vi "PCO_SensorInfo.vi"() -> (1 "Raw_Length":u16, 4 "Length":u16, 6 "PCO_SensorInfo_Raw_x64":T1, 7 "PCO_SensorInfo_Raw_win32":T2, 8 "PCO_SensorInfo":T3 {"iSensorInfoBits" items=["CONVERT_SENSOR_COLORIMAGE"=1, "CONVERT_SENSOR_UPPERALIGNED"=2]})   [LabVIEW 2019, in "Convert.lvlib"]
doc: "Use this template to build a VI to use as a subVI."
uses:
  Convert.lvlib
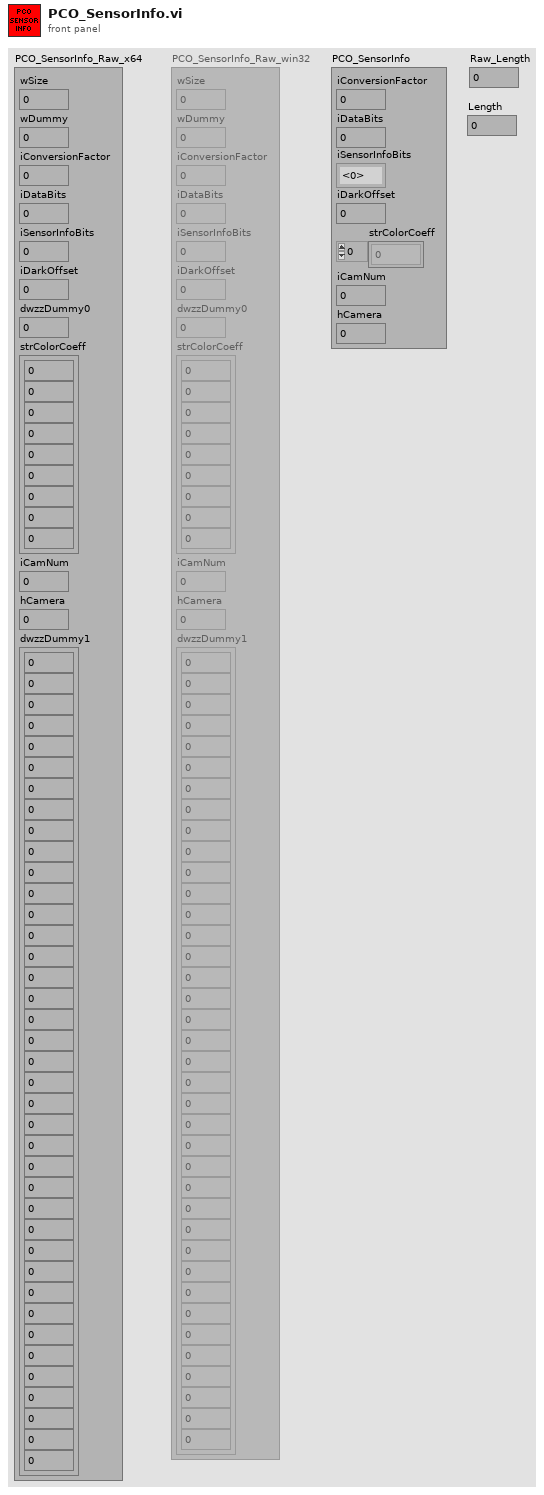
[diagram p1: front panel]
types:
  T1 = cluster{"wSize":u16, "wDummy":u16, "iConversionFactor":i32, "iDataBits":i32, "iSensorInfoBits":i32, "iDarkOffset":i32, "dwzzDummy0":u32, "strColorCoeff":cluster{dbl, dbl, dbl, dbl, dbl, dbl, dbl, dbl, dbl}, "iCamNum":i32, "hCamera":u64, "dwzzDummy1":cluster{u32, u32, u32, u32, u32, u32, u32, u32, u32, u32, u32, u32, u32, u32, u32, u32, u32, u32, u32, u32, u32, u32, u32, u32, u32, u32, u32, u32, u32, u32, u32, u32, u32, u32, u32, u32, u32, u32, u32}}
  T2 = cluster{"wSize":u16, "wDummy":u16, "iConversionFactor":i32, "iDataBits":i32, "iSensorInfoBits":i32, "iDarkOffset":i32, "dwzzDummy0":u32, "strColorCoeff":cluster{dbl, dbl, dbl, dbl, dbl, dbl, dbl, dbl, dbl}, "iCamNum":i32, "hCamera":u32, "dwzzDummy1":cluster{u32, u32, u32, u32, u32, u32, u32, u32, u32, u32, u32, u32, u32, u32, u32, u32, u32, u32, u32, u32, u32, u32, u32, u32, u32, u32, u32, u32, u32, u32, u32, u32, u32, u32, u32, u32, u32, u32}}
  T3 = cluster{"iConversionFactor":i32, "iDataBits":i32, "iSensorInfoBits":i32, "iDarkOffset":i32, "strColorCoeff":dbl[], "iCamNum":i32, "hCamera":u64}
  T4 = cluster{dbl, dbl, dbl, dbl, dbl, dbl, dbl, dbl, dbl}
  T5 = cluster{u32, u32, u32, u32, u32, u32, u32, u32, u32, u32, u32, u32, u32, u32, u32, u32, u32, u32, u32, u32, u32, u32, u32, u32, u32, u32, u32, u32, u32, u32, u32, u32, u32, u32, u32, u32, u32, u32, u32}
  T6 = cluster{u32, u32, u32, u32, u32, u32, u32, u32, u32, u32, u32, u32, u32, u32, u32, u32, u32, u32, u32, u32, u32, u32, u32, u32, u32, u32, u32, u32, u32, u32, u32, u32, u32, u32, u32, u32, u32, u32}
  T7 = enum8{"Enabled", "Disabled", "Disabled and Grayed Out"}
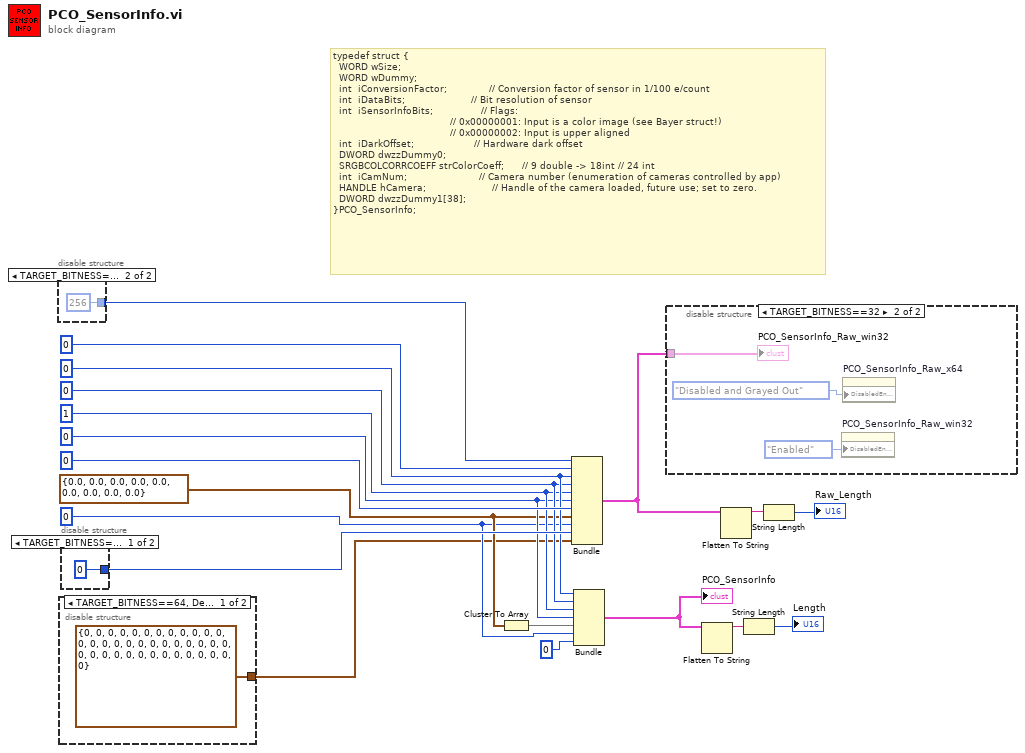
[diagram p0: block diagram]
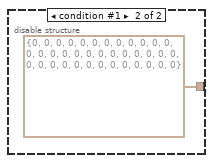
[diagram p2: hidden frame]
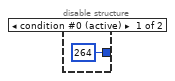
[diagram p3: hidden frame]
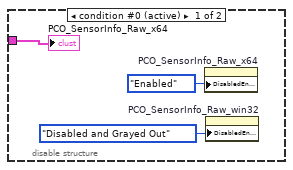
[diagram p4: hidden frame]
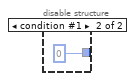
[diagram p5: hidden frame]
diagram:
  w5 = 0 ("iCamNum")
  w7 = T4 {0.0, 0.0, 0.0, 0.0, 0.0, 0.0, 0.0, 0.0, 0.0} ("strColorCoeff")
  w8 = 0 ("iDarkOffset")
  w9 = 1 ("iSensorInfoBits")
  w10 = 0 ("iDataBits")
  w11 = 0 ("iConversionFactor")
  # "typedef struct {\n  WORD wSize;\n  WORD wDummy;\n  int  iConversionFactor;              // Conversion factor of sensor in 1/100 e/count\n  int  iDataBits;                      // Bit resolution of sensor\n  int  iSensorInfoBits;                // Flags:\n                                       // 0x00000001: Input is a color image (see Bayer struct!)\n                                       // 0x00000002: Input is upper aligned\n  int  iDarkOffset;                    // Hardware dark offset\n  DWORD dwzzDummy0;                    \n  SRGBCOLCORRCOEFF strColorCoeff;      // 9 double -> 18int // 24 int\n  int  iCamNum;                        // Camera number (enumeration of cameras controlled by app)\n  HANDLE hCamera;                      // Handle of the camera loaded, future use; set to zero.\n  DWORD dwzzDummy1[38];\n}PCO_SensorInfo;"
  n1 = disable-structure "Diagram Disable Structure" shown="TARGET_BITNESS==32" {
    disable-tunnel: [u16 264 ("wSize") u16 256 ("wSize")] -> w2
    frame condition #0 (active) {
    }
    frame condition #1 {
    }
  }
  n2 = disable-structure "Diagram Disable Structure" shown="TARGET_BITNESS==64, Default" {
    disable-tunnel: [T5 {0, 0, 0, 0, 0, 0, 0, 0, 0, 0, 0, 0, 0, 0, 0, 0, 0, 0, 0, 0, 0, 0, 0, 0, 0, 0, 0, 0, 0, 0, 0, 0, 0, 0, 0, 0, 0, 0, 0} ("dwzzDummy1") T6 {0, 0, 0, 0, 0, 0, 0, 0, 0, 0, 0, 0, 0, 0, 0, 0, 0, 0, 0, 0, 0, 0, 0, 0, 0, 0, 0, 0, 0, 0, 0, 0, 0, 0, 0, 0, 0, 0} ("dwzzDummy1")] -> w1
    frame condition #0 (active) {
    }
    frame condition #1 {
    }
  }
  n3 = disable-structure "Diagram Disable Structure" shown="TARGET_BITNESS==64, Default" {
    disable-tunnel: [u64 0 ("hCamera") u32 0 ("hCamera")] -> w12
    frame condition #0 (active) {
    }
    frame condition #1 {
    }
  }
  n4 = Cluster To Array(cluster=w7) -> (array=w6:dbl[])
  n5 = Bundle("wSize"=w2, "wDummy"=u16 0, "iConversionFactor"=w11, "iDataBits"=w10, "iSensorInfoBits"=w9, "iDarkOffset"=w8, "dwzzDummy0"=u32 0, "strColorCoeff"=w7, "iCamNum"=w5, "hCamera"=w12, "dwzzDummy1"=w1) -> (w3:T1)  [unwired: 1 in]
  n6 = Bundle("iConversionFactor"=w11, "iDataBits"=w10, "iSensorInfoBits"=w9, "iDarkOffset"=w8, "strColorCoeff"=w6, "iCamNum"=w5, "hCamera"=u64 0) -> (w19:T3)  [unwired: 1 in]
  "PCO_SensorInfo" <- w19
  n7 = disable-structure "Diagram Disable Structure" shown="TARGET_BITNESS==32" {
    disable-tunnel: w3 -> [w27 w31]
    frame condition #0 (active) {
      n8 = property on="PCO_SensorInfo_Raw_x64" class="Clust (strict)"("DisabledEnum"=T7."Enabled" ("Disabled")) -> ()  [unwired: 2 in, 2 out]
      n9 = property on="PCO_SensorInfo_Raw_win32" class="Clust (strict)"("DisabledEnum"=T7."Disabled and Grayed Out" ("Disabled")) -> ()  [unwired: 2 in, 2 out]
      "PCO_SensorInfo_Raw_x64" <- w27
    }
    frame condition #1 {
      n10 = property on="PCO_SensorInfo_Raw_win32" class="Clust (strict)"("DisabledEnum"=T7."Enabled" ("Disabled")) -> ()  [unwired: 2 in, 2 out]
      n11 = property on="PCO_SensorInfo_Raw_x64" class="Clust (strict)"("DisabledEnum"=T7."Disabled and Grayed Out" ("Disabled")) -> ()  [unwired: 2 in, 2 out]
      "PCO_SensorInfo_Raw_win32" <- w31
    }
  }
  n12 = Flatten To String(anything=w19) -> (data string=w18:string)  [unwired: 3 in, 2 out]
  n13 = Flatten To String(anything=w3) -> (data string=w17:string)  [unwired: 3 in, 2 out]
  n14 = String Length(string=w18) -> (length=→"Length":i32)
  n15 = String Length(string=w17) -> (length=→"Raw_Length":i32)
